vi "3.Bounce Window_Log On&Exit.vi"(11 "群組：":T1) -> (3 "登出/離開":T2)   [LabVIEW 2015]
uses:
  0.Main_Control/Control_Bounce Window_Main_Log On-Exit.ctl
  <vilib>/Utility/miscctls.llb/LVPointTypeDef.ctl
panel:
  in  "離開":bool
  in  "使用者登出":bool
  in  "關機":bool
  in  "回到作業系統":bool
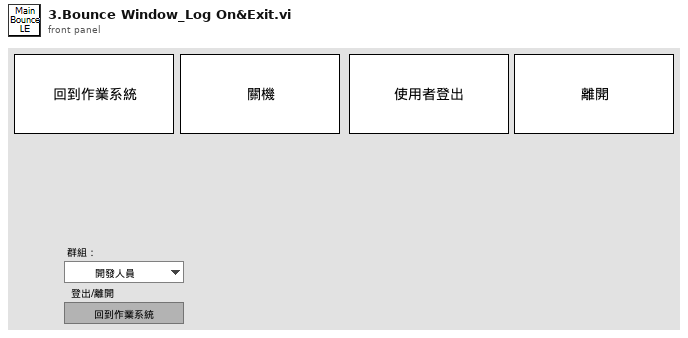
[diagram p1: front panel]
types:
  T1 = typedef "Control_User account_Permissions.ctl" = enum16{"開發人員", "管理者", "工程師", "作業員"}
  T2 = typedef "Control_Bounce Window_Main_Log On-Exit.ctl" = enum16{"回到作業系統", "關機", "使用者登出", "離開", "等待"}
  T3 = typedef "LVPointTypeDef.ctl" = cluster{"Horizontal":i16, "Vertical":i16}
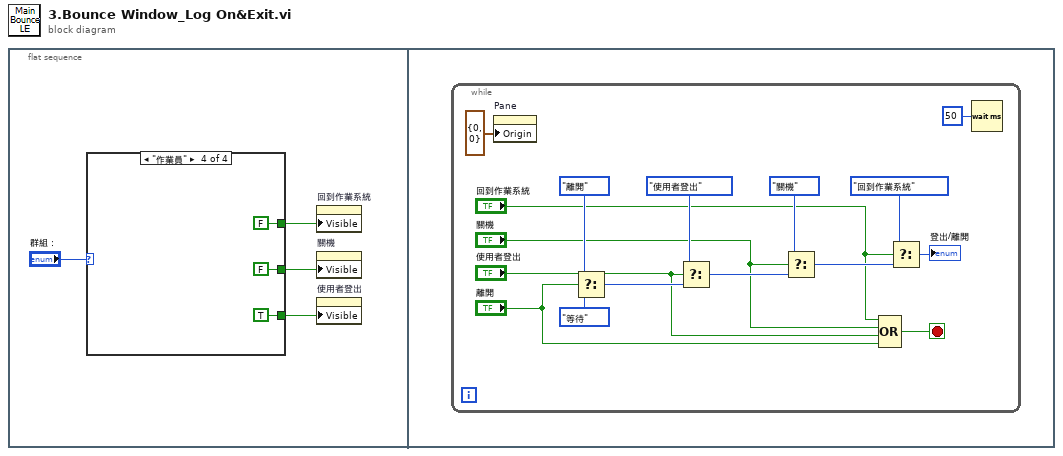
[diagram p0: block diagram]
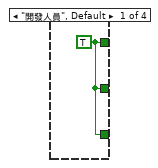
[diagram p2: hidden frame]
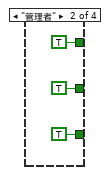
[diagram p3: hidden frame]
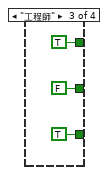
[diagram p4: hidden frame]
diagram:
  n1 = flat-sequence {
    frame #0 {
      n2 = case shown="\"作業員\"" "群組：" {
        tunnel: [w5 TRUE TRUE TRUE] -> w4
        tunnel: [w5 TRUE TRUE FALSE] -> w2
        tunnel: [w5 TRUE FALSE FALSE] -> w3
        frame "開發人員", Default {
          w5 = TRUE
        }
        frame "管理者" {
        }
        frame "工程師" {
        }
        frame "作業員" {
        }
      }
      n3 = property on="回到作業系統" class="Bool"("Visible"=w2) -> ()  [unwired: 2 in, 2 out]
      n4 = property on="關機" class="Bool"("Visible"=w3) -> ()  [unwired: 2 in, 2 out]
      n5 = property on="使用者登出" class="Bool"("Visible"=w4) -> ()  [unwired: 2 in, 2 out]
    }
    frame #1 {
      n6 = while {
        stop <- w17 stop-if-true
        n7 = property on="Pane" class="Pane"("Origin"=T3 {"Horizontal"=0, "Vertical"=0}) -> ()  [unwired: 2 in, 2 out]
        n8 = Select(t=Control_Bounce_Window_Main_Log_On-Exit."離開" ("登出/離開"), s="離開", f=Control_Bounce_Window_Main_Log_On-Exit."等待" ("登出/離開")) -> (s? t:f=w27:T2)
        n9 = Select(t=Control_Bounce_Window_Main_Log_On-Exit."使用者登出" ("登出/離開"), s="使用者登出", f=w27) -> (s? t:f=w25:T2)
        n10 = Select(t=Control_Bounce_Window_Main_Log_On-Exit."關機" ("登出/離開"), s="關機", f=w25) -> (s? t:f=w22:T2)
        n11 = Compound Arithmetic op=OR("回到作業系統", "關機", "使用者登出", "離開") -> (w17:bool)
        n12 = Select(t=Control_Bounce_Window_Main_Log_On-Exit."回到作業系統" ("登出/離開"), s="回到作業系統", f=w22) -> (s? t:f=→"登出/離開":T2)
        n13 = Wait (ms)(milliseconds to wait=u32 50) -> ()  [unwired: 1 out]
      }
    }
  }
